vi "AMPL_OFFSET(LTE).vi"(0 "Session In":refnum<visa-resource-name>="TCPIP0::K-N90X0A-00005.local::hislip0::INSTR", 2 "Gain(dB)":dbl=1.0, 11 "error in":errorcluster {"code" format="%.0x"}, 12 "BTS/MS":string(combo)="BTS", 13 "Timeout":u32=3000, 14 "R/W":u16(ring) items=["WO"=2, "RO"=1, "R/W"=0]) -> (4 "Session Out":refnum<visa-resource-name>, 8 "Gain":dbl, 15 "error out":errorcluster {"code" format="%.0x"})   [LabVIEW 2018]
doc: "Launches the Instrument I/O Assistant, which you can use to communicate with message-based instruments and graphically parse the response. For example you can communicate with an instrument that uses a serial, Ethernet, or GPIB interface."
panel:
  # "Adds loss to the measurement\nUse a loss (-dB)  to apply + correction\ne.g. -1 will add 1 to the result"
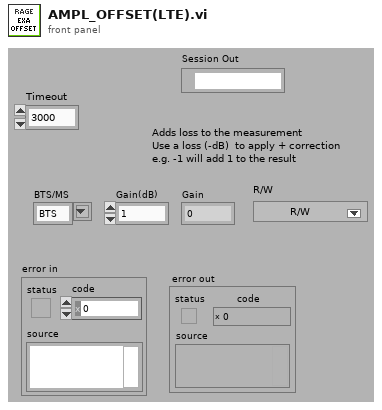
[diagram p1: front panel]
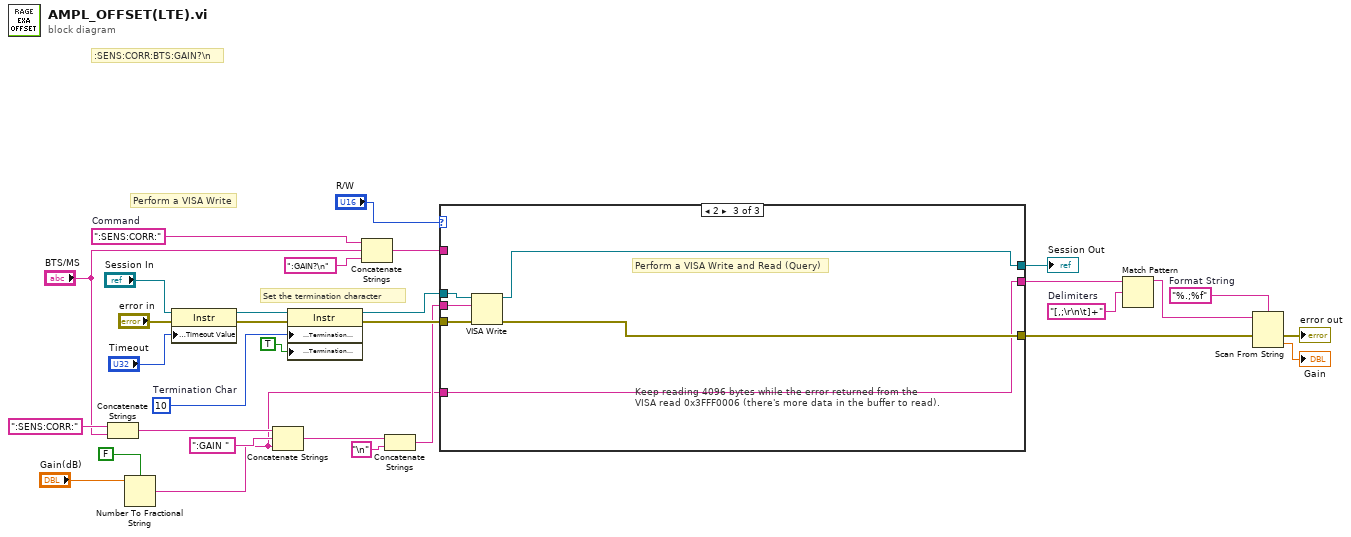
[diagram p0: block diagram]
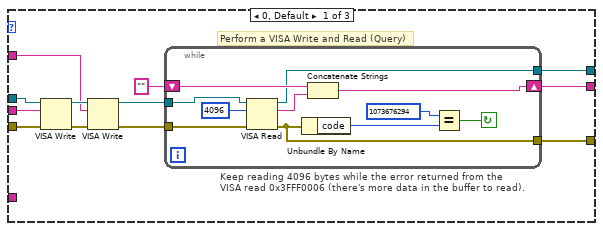
[diagram p2: hidden frame]
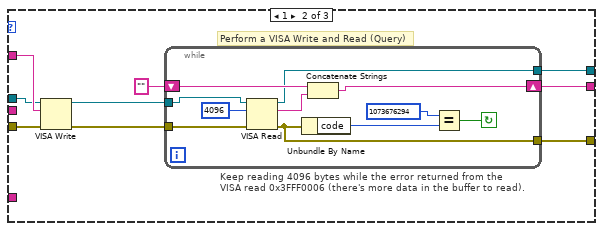
[diagram p3: hidden frame]
diagram:
  w11 = "[,;\r\n\t]+"  # Delimiters
  w14 = "%.;%f"  # Format String
  w8 = ":SENS:CORR:"  # Command
  w25 = u8 10  # Termination Char
  # ":SENS:CORR:BTS:GAIN?\\n"
  # "Perform a VISA Write"
  # "Set the termination character"
  n1 = Concatenate Strings(":SENS:CORR:" ("staticText"), "BTS/MS") -> (w6:string)
  n2 = Number To Fractional String(use system decimal point (T)=FALSE, number="Gain(dB)") -> (F-format string=w1:string)  [unwired: 2 in]
  n3 = property class="Instr"(reference="Session In", error in="error in", "General Settings:Timeout Value"="Timeout") -> (reference out=w24:refnum<visa-resource-name>, error out=w27:errorcluster)
  n4 = Concatenate Strings(w6, ":GAIN " ("staticText"), w1) -> (w19:string)
  n5 = property class="Instr"(reference=w24, error in=w27, "Message Based Settings:Termination Character"=w25, "Message Based Settings:Termination Character Enable"=TRUE ("enable")) -> (reference out=w10:refnum<visa-resource-name>, error out=w26:errorcluster)
  n6 = Concatenate Strings(w8, "BTS/MS", ":GAIN?\n") -> (w5:string)
  n7 = Concatenate Strings(w19, "\n" ("StaticText")) -> (w20:string)
  n8 = case shown="2" "R/W" {
    tunnel: w26 -> [w43 w56 w80]
    tunnel: w20 -> [w41 _ w79]
    tunnel: [w38 w61 w76] -> w17
    tunnel: [w36 w59 w75] -> w16
    tunnel: w10 -> [w35 w55 w78]
    tunnel: [w34 w58 w77] -> w9
    tunnel: w5 -> [w32 w57 _]
    tunnel: w1 -> [_ _ w75]
    frame 0, Default {
      # "Perform a VISA Write and Read (Query)"
      # "Keep reading 4096 bytes while the error returned from the\nVISA read 0x3FFF0006 (there's more data in the buffer to read)."
      n9 = VISA Write(VISA resource name=w35, write buffer=w41, error in (no error)=w43) -> (VISA resource name out=w33:refnum<visa-resource-name>, error out=w42:errorcluster)  [unwired: 1 out]
      n10 = VISA Write(VISA resource name=w33, write buffer=w32, error in (no error)=w42) -> (VISA resource name out=w40:refnum<visa-resource-name>, error out=w39:errorcluster)  [unwired: 1 out]
      n11 = while {
        tunnel: w40 -> [w51]
        shift-right: [w45] -> w36
        shift-left: "" -> [w50]
        tunnel: w39 -> [w48]
        tunnel: [w47] -> w38
        tunnel: [w44] -> w34
        stop <- w46 continue-if-true
        n12 = VISA Read(VISA resource name=w51, byte count=u32 4096 ("byte count (0)"), error in (no error)=w48) -> (VISA resource name out=w44:refnum<visa-resource-name>, read buffer=w49:string, error out=w47:errorcluster)  [unwired: 1 out]
        n13 = Unbundle By Name(w47) -> ("code"=w53:i32)
        n14 = Concatenate Strings(w50, w49) -> (w45:string)
        n15 = Equal?(x=1073676294, y=w53) -> (x = y?=w46:bool)
      }
    }
    frame 1 {
      # "Perform a VISA Write and Read (Query)"
      # "Keep reading 4096 bytes while the error returned from the\nVISA read 0x3FFF0006 (there's more data in the buffer to read)."
      n16 = VISA Write(VISA resource name=w55, write buffer=w57, error in (no error)=w56) -> (VISA resource name out=w63:refnum<visa-resource-name>, error out=w62:errorcluster)  [unwired: 1 out]
      n17 = while {
        tunnel: w63 -> [w71]
        shift-right: [w65] -> w59
        shift-left: "" -> [w70]
        tunnel: w62 -> [w68]
        tunnel: [w67] -> w61
        tunnel: [w64] -> w58
        stop <- w66 continue-if-true
        n18 = VISA Read(VISA resource name=w71, byte count=u32 4096 ("byte count (0)"), error in (no error)=w68) -> (VISA resource name out=w64:refnum<visa-resource-name>, read buffer=w69:string, error out=w67:errorcluster)  [unwired: 1 out]
        n19 = Unbundle By Name(w67) -> ("code"=w73:i32)
        n20 = Concatenate Strings(w70, w69) -> (w65:string)
        n21 = Equal?(x=1073676294, y=w73) -> (x = y?=w66:bool)
      }
    }
    frame 2 {
      # "Perform a VISA Write and Read (Query)"
      # "Keep reading 4096 bytes while the error returned from the\nVISA read 0x3FFF0006 (there's more data in the buffer to read)."
      n22 = VISA Write(VISA resource name=w78, write buffer=w79, error in (no error)=w80) -> (VISA resource name out=w77:refnum<visa-resource-name>, error out=w76:errorcluster)  [unwired: 1 out]
    }
  }
  "Session Out" <- w9
  n23 = Match Pattern(string=w16, regular expression=w11) -> (before substring=w15:string)  [unwired: 1 in, 3 out]
  n24 = Scan From String(format string=w14, input string=w15, error in=w17) -> (error out=→"error out":errorcluster, output 1=→"Gain":dbl)  [unwired: 2 in, 2 out]
